vi "Position_Based_L4_Motion.vi"(8 "assign z":dbl, 9 "EyeCenter x val":dbl, 10 "current z":dbl, 11 "current x":dbl) -> (3 "L4 motion (cnts)":i32)   [LabVIEW 2010]
doc: "This VI calculates the L4 motion based on the current (x,~,z) position.\nIt is designed so that the aspiration hole is always facing towards a virtual axis (EyeCenter x val,~,assign z)."
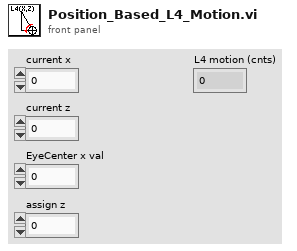
[diagram p1: front panel]
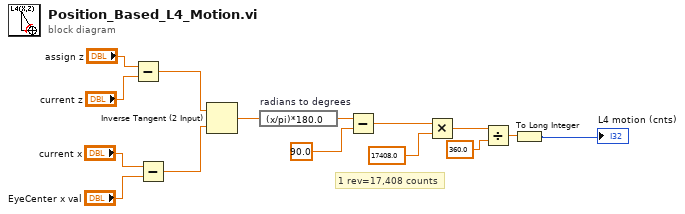
[diagram p0: block diagram]
diagram:
  # "1 rev=17,408 counts"
  n1 = Subtract(x="assign z", y="current z") -> (x-y=w11:dbl)
  n2 = Subtract(x="current x", y="EyeCenter x val") -> (x-y=w10:dbl)
  n3 = Inverse Tangent (2 Input)(1:w10, 2:w11) -> (0:w9:dbl)
  n4 = expression code="(x/pi)*180.0" "radians to degrees"(w9) -> (w8:dbl)
  n5 = Subtract(x=w8, y=90.0) -> (x-y=w2:dbl)
  n6 = Multiply(x=w2, y=17408.0) -> (x*y=w3:dbl)
  n7 = Divide(x=w3, y=360.0) -> (x/y=w6:dbl)
  n8 = To Long Integer(number=w6) -> (32bit integer=→"L4 motion (cnts)":i32)
